vi "430_TCP_Open.vi"(0 "IP Address":string, 3 "timeout ms (2000)":i32=2000, 5 "error in (no error)":errorcluster) -> (6 "connection ID":refnum<k5>, 7 "Init Response":string, 8 "error out":errorcluster)   [LabVIEW 2011]
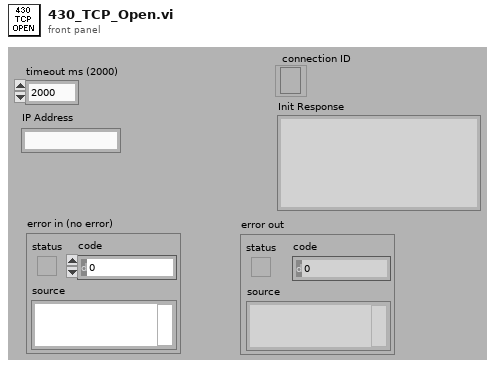
[diagram p1: front panel]
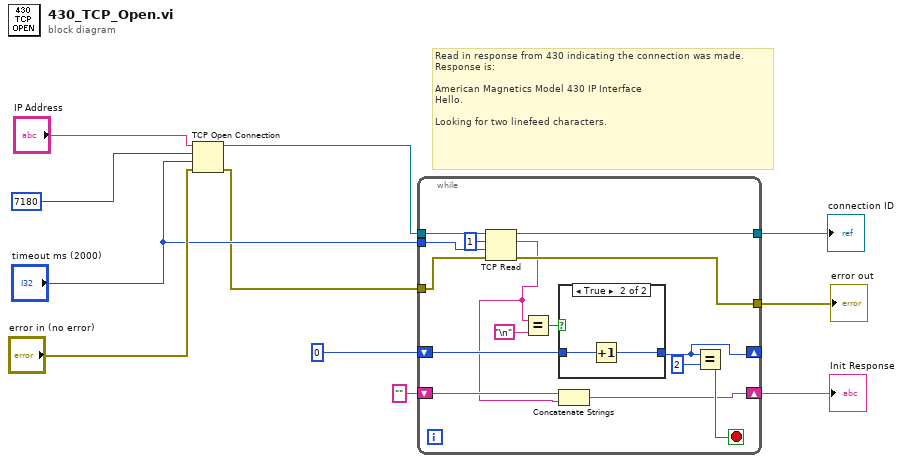
[diagram p0: block diagram]
diagram:
  # "Read in response from 430 indicating the connection was made.\nResponse is:\n\nAmerican Magnetics Model 430 IP Interface\nHello.\n\nLooking for two linefeed characters."
  n1 = TCP Open Connection(address="IP Address", remote port or service name=u16 7180, timeout ms (60000)="timeout ms (2000)", error in (no error)="error in (no error)") -> (connection ID=w9:refnum<k5>, error out=w5:errorcluster)  [unwired: 1 in]
  n2 = while {
    tunnel: w9 -> [w26]
    tunnel: [w25] -> w8
    tunnel: "timeout ms (2000)" -> [w23]
    tunnel: w5 -> [w22]
    tunnel: [w21] -> w4
    shift-right: [w14] -> w2
    shift-left: "" -> [w15]
    shift-right: [w12] -> _
    shift-left: 0 -> [w20]
    stop <- w18 stop-if-true
    n3 = TCP Read(connection ID=w26, bytes to read=1, error in (no error)=w22, 9:w23) -> (connection ID out=w25:refnum<k5>, data out=w13:string, error out=w21:errorcluster)  [unwired: 1 in]
    n4 = Equal?(x=w13, y="\n") -> (x = y?=w17:bool)
    n5 = case shown="True" w17 {
      tunnel: w20 -> [w27 w29]
      tunnel: [w27 w28] -> w12
      frame False {
      }
      frame True {
        n6 = Increment(x=w29) -> (x+1=w28:i32)
      }
    }
    n7 = Concatenate Strings(w15, w13) -> (w14:string)
    n8 = Equal?(x=w12, y=2) -> (x = y?=w18:bool)
  }
  "error out" <- w4
  "connection ID" <- w8
  "Init Response" <- w2
